vi "topic_to_Array.vi"(11 "Topic":string) -> (3 "Topic (Array)":string[](array[string]))   [LabVIEW 2017]
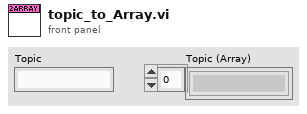
[diagram p1: front panel]
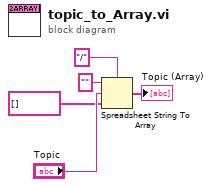
[diagram p0: block diagram]
diagram:
  n1 = Spreadsheet String To Array(delimiter (Tab)="/" ("string"), format string="", spreadsheet string="Topic", array type (2D Dbl)=string[] []) -> (array=→"Topic (Array)":string[])
